vi "enum to code.vi"(11 "file error":T1) -> (3 "code":i32)   [LabVIEW 2013, in "file errors.lvlib"]
uses:
  file errors.lvlib
  file error.ctl
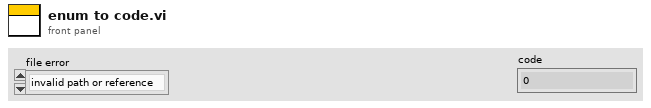
[diagram p1: front panel]
types:
  T1 = typedef "file errors.lvlib/file error.ctl" = enum16{"invalid path or reference", "end of file", "file already opened", "generic file error", "file not found", "permissions invalid", "disk full", "duplicate path", "too many open file handles", "useless generic error"}
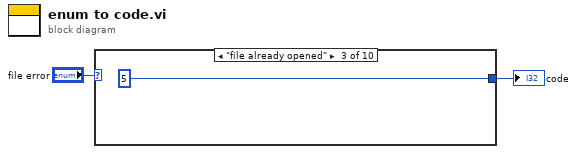
[diagram p0: block diagram]
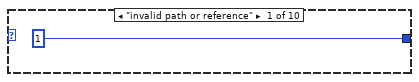
[diagram p2: hidden frame]
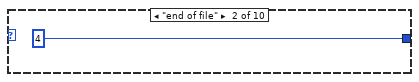
[diagram p3: hidden frame]
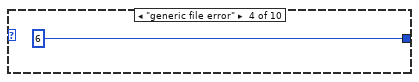
[diagram p4: hidden frame]
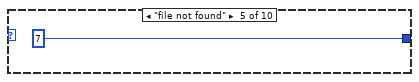
[diagram p5: hidden frame]
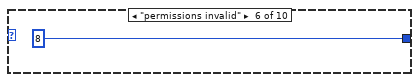
[diagram p6: hidden frame]
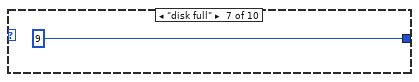
[diagram p7: hidden frame]
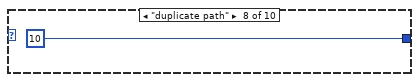
[diagram p8: hidden frame]
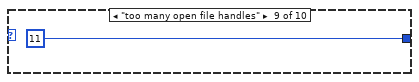
[diagram p9: hidden frame]
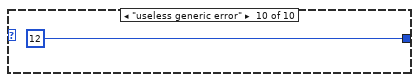
[diagram p10: hidden frame]
diagram:
  n1 = case shown="\"file already opened\"" "file error" {
    tunnel: [1 4 5 6 7 8 9 10 11 12] -> w1
    frame "invalid path or reference" {
    }
    frame "end of file" {
    }
    frame "file already opened" {
    }
    frame "generic file error" {
    }
    frame "file not found" {
    }
    frame "permissions invalid" {
    }
    frame "disk full" {
    }
    frame "duplicate path" {
    }
    frame "too many open file handles" {
    }
    frame "useless generic error" {
    }
  }
  "code" <- w1
